vi "Global Shutter.vi"() -> ()   [LabVIEW 2014]
panel:
  out "Error Out":errorcluster
  in  "VISA Refnum out":refnum<visa-resource-name>
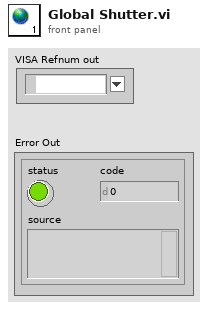
[diagram p1: front panel]
diagram:
